vi "Remove RTV [by older scope].vi"(0 "RT Variables in":refnum<class "RT Variables.lvclass">, 5 "RTV Scope":i64, 11 "error in (no error)":errorcluster) -> (4 "RT Variables out":refnum<class "RT Variables.lvclass">, 15 "error out":errorcluster)   [LabVIEW 2019, in "LSL.lvlib" / "RT Variables.lvclass"]
uses:
  RT Variables.lvclass
  RT Variables.lvclass/RT Variables.ctl
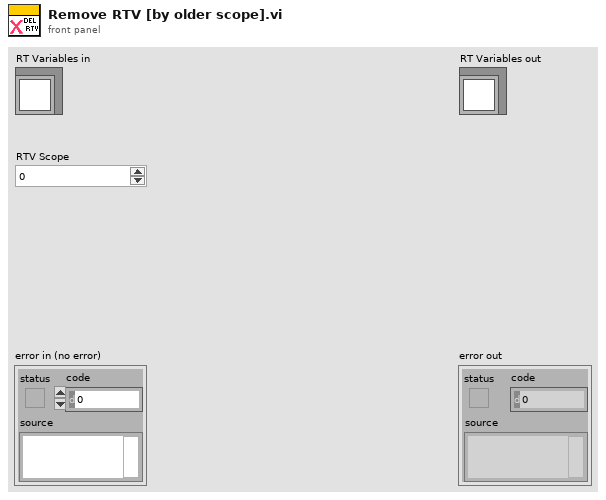
[diagram p1: front panel]
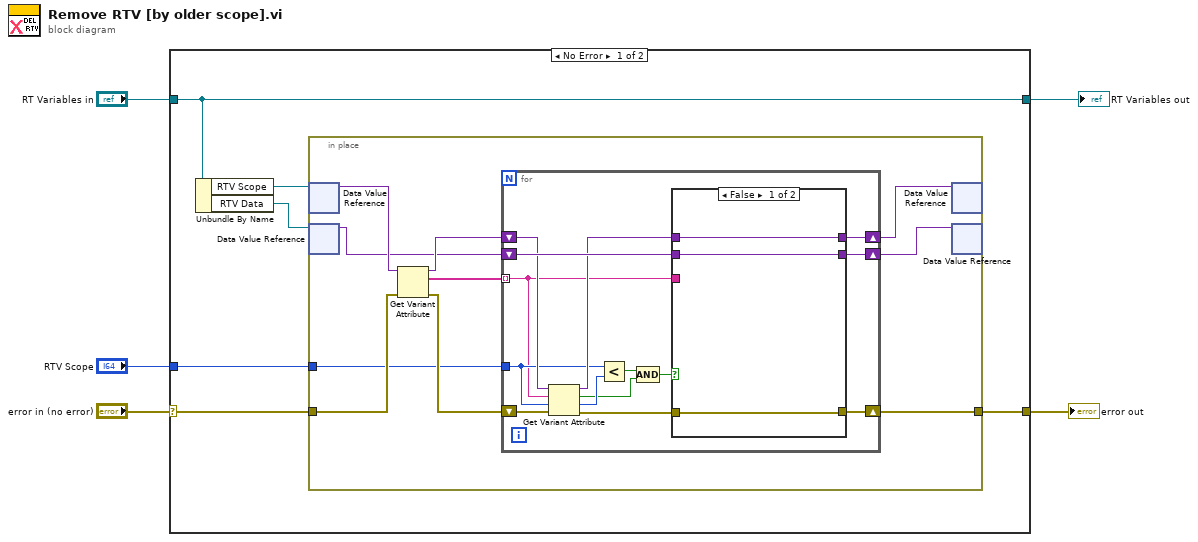
[diagram p0: block diagram]
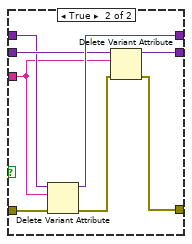
[diagram p2: hidden frame]
diagram:
  n1 = case shown="No Error" "error in (no error)" {
    selector: "error in (no error)" -> [w11 w48]
    tunnel: [w10 w48] -> w4
    tunnel: "RTV Scope" -> [w9 _]
    tunnel: "RT Variables in" -> [w6 w47]
    tunnel: [w6 w47] -> w1
    frame No Error {
      n2 = Unbundle By Name(w6) -> ("RTV Scope"=w8:refnum<data-value>, "RTV Data"=w7:refnum<data-value>)
      n3 = in-place {
        in-place-border: w11 -> [w21]
        in-place-border: [w20] -> w10
        in-place-border: w9 -> [w16]
        n4 = in-place-dvr #1(w8) -> (w15:variant)  [unwired: 1 out]
        n5 = in-place-dvr #2(w7) -> (w13:variant)  [unwired: 1 out]
        n6 = Get Variant Attribute(Variant=w15, error in=w21) -> (duplicate Variant=w17:variant, names=w18:string[], error out=w19:errorcluster)  [unwired: 2 in, 1 out]
        n7 = for {
          shift-right: [w35] -> w14
          shift-left: w17 -> [w31]
          shift-right: [w33] -> w12
          shift-left: w13 -> [w34]
          shift-right: [w29] -> w20
          shift-left: w19 -> [w32]
          tunnel: w18 -> [w22] mode=indexing
          tunnel: w16 -> [w28]
          n8 = Get Variant Attribute(Variant=w31, name=w22, default value (empty Variant)=w28, error in=w32) -> (duplicate Variant=w30:variant, found=w25:bool, value=w27:i64, error out=w24:errorcluster)
          n9 = Less?(x=w28, y=w27) -> (x < y?=w26:bool)
          n10 = Compound Arithmetic op=AND(w26, w25) -> (w23:bool)
          n11 = case shown="False" w23 {
            tunnel: [w36 w46] -> w35
            tunnel: w34 -> [w37 w45]
            tunnel: [w37 w44] -> w33
            tunnel: w30 -> [w36 w43]
            tunnel: [w38 w41] -> w29
            tunnel: w24 -> [w38 w40]
            tunnel: w22 -> [_ w39]
            frame False {
            }
            frame True {
              n12 = Delete Variant Attribute(4:w40, 6:w39, 7:w43) -> (0:w42:errorcluster, 3:w46:variant)  [unwired: 1 out]
              n13 = Delete Variant Attribute(4:w42, 6:w39, 7:w45) -> (0:w41:errorcluster, 3:w44:variant)  [unwired: 1 out]
            }
          }
        }
        n14 = in-place-dvr #1(w14) -> ()  [unwired: 2 out]
        n15 = in-place-dvr #2(w12) -> ()  [unwired: 2 out]
      }
    }
    frame Error {
    }
  }
  "error out" <- w4
  "RT Variables out" <- w1
